vi "TwGetBufTimeFromShMem.vi"(2 "WriteIndex":i32, 3 "BufIndex":i32, 4 "error in (no error)":errorcluster) -> (0 "BufTime":dbl, 1 "error out":errorcluster)   [LabVIEW 2009]
uses:
  TofDaqDll.dll
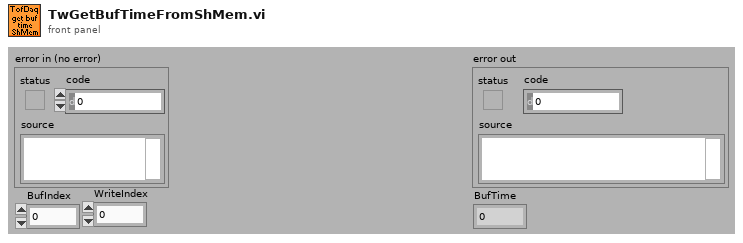
[diagram p1: front panel]
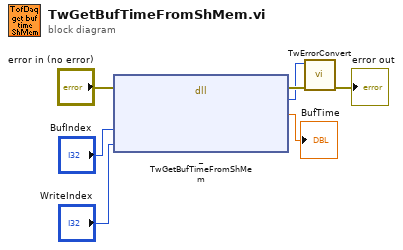
[diagram p0: block diagram]
diagram:
  n1 = dll-call lib="C:/Users/TofEmp/Desktop/LVTest/TofDaqDll.dll" fn="_TwGetBufTimeFromShMem"(error in="error in (no error)", "BufIndex"="BufIndex", "WriteIndex"="WriteIndex") -> (error out=w6:errorcluster, "TwRetVal"=w4:i32, "BufTime"=→"BufTime":dbl)  [unwired: 4 in, 2 out]
  n2 = call "TwErrorConvert.vi"("error in (no error)"=w6, "error code"=w4) -> ("error out"=→"error out":errorcluster)  [unwired: 9 out]
